vi "Rx Channel Config Page.vi"(8 "error in (no error)":errorcluster, 11 "Node Ptr":T1 format="%.0x") -> (0 "error out":errorcluster)   [LabVIEW 2016, in "UDP-Custom-Device System Explorer.lvlib"]
uses:
  UDP-Custom-Device System Explorer.lvlib
  <vilib>/NI Veristand/Custom Device API/Custom Device Item Ref.ctl
  <vilib>/NI VeriStand/Custom Device API/Custom Device API.lvlib
  Property Accessors/Shared Channel Accessors.lvlib
  <vilib>/NI VeriStand/Custom Device Tools/Custom Device Utility Library/Custom Device Utility Library.lvlib
panel:
  out "Imported Channel Configuration":i32[](listbox) caption="Channels"
  in  "Channel Configuration File":path
  in  "Description":string
  out "Name":string
  in  "SHDocVw.IWebBrowser":refnum<k7>(container)
  in  "General Header":cluster{"Section Name":string}={"Section Name"="Channel Configuration"}
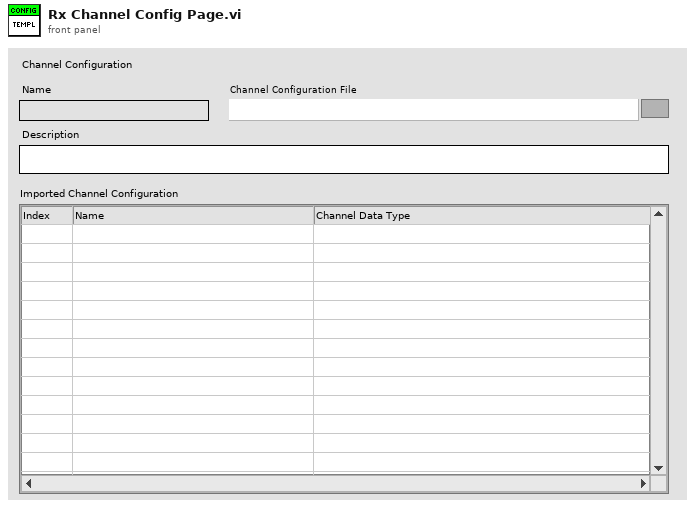
[diagram p1: front panel]
types:
  T1 = typedef "Custom Device API.lvlib/Custom Device Item Ref.ctl" = u64
  T2 = typedef "Custom Device API.lvlib/Custom Device Commands.ctl" = enum16{"Default", "Item renamed", "Shutdown", "Dynamic button pressed"}
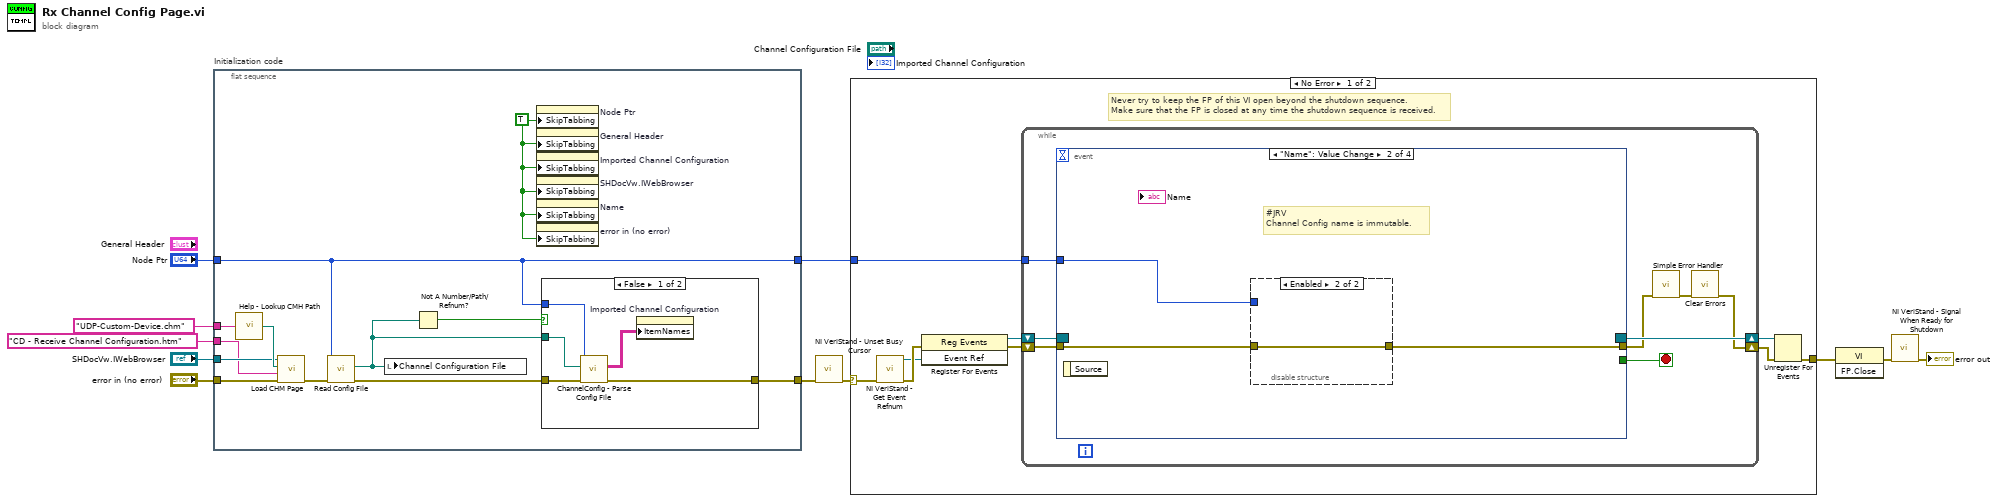
[diagram p0: block diagram]
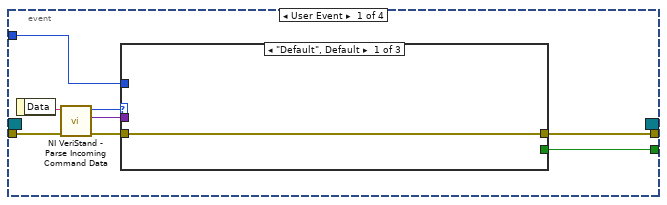
[diagram p3: hidden frame]
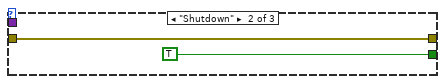
[diagram p4: hidden frame]
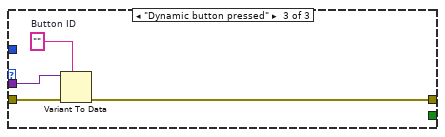
[diagram p5: hidden frame]
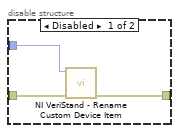
[diagram p6: hidden frame]
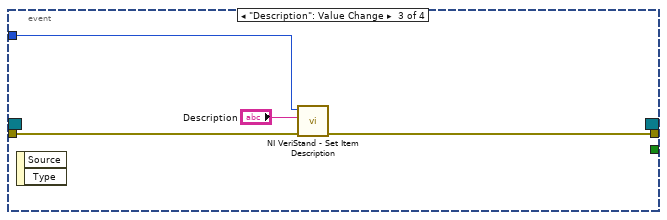
[diagram p7: hidden frame]
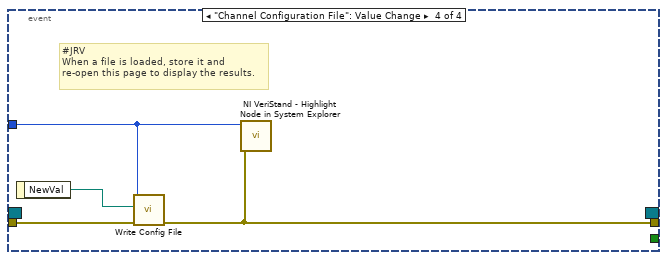
[diagram p8: hidden frame]
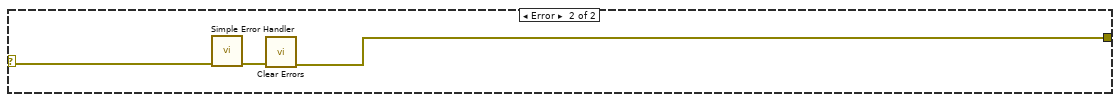
[diagram p9: hidden frame]
diagram:
  n1 = flat-sequence "Initialization code" {
    tunnel: "error in (no error)" -> [w22]
    tunnel: "Node Ptr" -> [w13]
    tunnel: [w17] -> w7
    tunnel: [w13] -> w4
    tunnel: "SHDocVw.IWebBrowser" -> [w21]
    tunnel: "CD - Receive Channel Configuration.htm" ("CD_CHM_Section") -> [w19]
    tunnel: "UDP-Custom-Device.chm" ("CD_CHM_FileName") -> [w20]
    frame #0 {
      w12 = TRUE ("Skip When Tabbing")
      n2 = call "Help - Lookup CMH Path.vi"("Main CMH File"=w20) -> ("Compiled CMH Path"=w23:path)
      n3 = call <vilib>:"Load CHM Page.vi"("error in (no error)"=w22, "HTML File"=w19, "Compiled CHM Path"=w23, "Web Browser Reference"=w21) -> ("error out"=w18:errorcluster)  [unwired: 7 in]
      n4 = call "Read Config File.vi"("error in (no error)"=w18, "Node Ptr"=w13) -> ("error out"=w16:errorcluster, "Config File"=w14:path)  [unwired: 7 in, 1 out]
      n5 = local write "Channel Configuration File"(w14) -> ()
      n6 = Not A Number/Path/Refnum?(number/path/refnum=w14) -> (NaN/Path/Refnum?=w15:bool)
      n7 = property on="Node Ptr" class="DigNum (strict)"("SkipTabbing"=w12) -> ()  [unwired: 2 in, 2 out]
      n8 = property on="General Header" class="Clust (strict)"("SkipTabbing"=w12) -> ()  [unwired: 2 in, 2 out]
      n9 = property on="Imported Channel Configuration" class="MCListbox (strict)"("SkipTabbing"=w12) -> ()  [unwired: 2 in, 2 out]
      n10 = property on="SHDocVw.IWebBrowser" class="AXCont"("SkipTabbing"=w12) -> ()  [unwired: 2 in, 2 out]
      n11 = property on="Name" class="Str"("SkipTabbing"=w12) -> ()  [unwired: 2 in, 2 out]
      n12 = property on="error in (no error)" class="Clust (strict)"("SkipTabbing"=w12) -> ()  [unwired: 2 in, 2 out]
      n13 = case shown="False" w15 {
        tunnel: [w25 w29] -> w17
        tunnel: w16 -> [w26 w29]
        tunnel: w14 -> [w28 _]
        tunnel: w13 -> [w27 _]
        frame False {
          n14 = call "ChannelConfig - Parse Config File.vi"("error in (no error)"=w26, "Config Path"=w28, "Node Ptr"=w27) -> ("error out"=w25:errorcluster, "Channel Configuration"=w24:string[][])  [unwired: 6 in, 1 out]
          n15 = property on="Imported Channel Configuration" class="MCListbox (strict)"("ItemNames"=w24) -> ()  [unwired: 2 in, 2 out]
        }
        frame True {
        }
      }
    }
  }
  n16 = call <vilib>:"NI VeriStand - Unset Busy Cursor.vi"("error in (no error)"=w7) -> ("error out"=w6:errorcluster)  [unwired: 10 out]
  n17 = case shown="No Error" w6 {
    selector: w6 -> [w30 w79]
    tunnel: [w35 w77] -> w11
    tunnel: w4 -> [w31 _]
    frame No Error {
      # "Never try to keep the FP of this VI open beyond the shutdown sequence.\nMake sure that the FP is closed at any time the shutdown sequence is received."
      n18 = call <vilib>:"NI VeriStand - Get Event Refnum.vi"("error in (no error)"=w30) -> ("error out"=w38:errorcluster, "Event Ref"=w34:refnum<user-event>)  [unwired: 9 out]
      n19 = register-events(error in=w38, w34) -> (reference out=w32:refnum<event-registration>, error out=w33:errorcluster)  [unwired: 1 in]
      n20 = while {
        tunnel: w31 -> [w42]
        shift-right: [w39] -> w36
        shift-left: w33 -> [w45]
        shift-right: [w46] -> w37
        shift-left: w32 -> [w44]
        stop <- w43 stop-if-true
        n21 = event shown="[1] \"Name\": Value Change" {
          selector: w44 -> [_ _ _ _]
          dyn-events: [_ _ _ _] -> w46
          timeout: _ -> [_ _ _ _]
          tunnel: w45 -> [w54 w64 w72 w74]
          tunnel: [w50 _ _ _] -> w43
          tunnel: [w49 w62 w69 w73] -> w41
          tunnel: w42 -> [w48 w63 w71 w76]
          event User Event {
            n22 = event-data() -> ("Data"=w53:string)  [unwired: 1 out]
            n23 = call <vilib>:"NI VeriStand - Parse Incoming Command Data.vi"("error in (no error)"=w54, "Incoming data"=w53) -> ("error out"=w52:errorcluster, "Outgoing data"=w47:variant, "Action"=w51:T2)  [unwired: 7 out]
            n24 = case shown="\"Default\", Default" w51 {
              tunnel: w52 -> [w55 w56 w61]
              tunnel: [_ TRUE _] -> w50
              tunnel: [w55 w56 w58] -> w49
              tunnel: w48 -> [_ _ _]
              tunnel: w47 -> [_ _ w60]
              frame "Default", Default {
              }
              frame "Shutdown" {
              }
              frame "Dynamic button pressed" {
                w59 = ""  # Button ID
                n25 = Variant To Data(error in=w61, type=w59, Variant=w60) -> (error out=w58:errorcluster)  [unwired: 1 out]
              }
            }
          }
          event "Name": Value Change {
            # "#JRV\nChannel Config name is immutable."
            n26 = event-data() -> ()  [unwired: 2 out]
            n27 = disable-structure shown="Enabled" {
              disable-tunnel: w64 -> [w67 w68]
              disable-tunnel: w63 -> [w66 _]
              disable-tunnel: [w65 w68] -> w62
              frame Disabled {
                n28 = call <vilib>:"NI VeriStand - Rename Custom Device Item.vi"("error in (no error)"=w67, "Item Ref in"=w66) -> ("error out"=w65:errorcluster)  [unwired: 7 in, 2 out]
              }
              frame Enabled {
              }
            }
          }
          event "Description": Value Change {
            n29 = event-data() -> ()  [unwired: 3 out]
            n30 = call <vilib>:"NI VeriStand - Set Item Description.vi"("error in (no error)"=w72, "Description"="Description", "Item Ref in"=w71) -> ("error out"=w69:errorcluster)  [unwired: 6 in, 2 out]
          }
          event "Channel Configuration File": Value Change {
            # "#JRV\nWhen a file is loaded, store it and\nre-open this page to display the results."
            n31 = event-data() -> ("NewVal"=w75:path)  [unwired: 1 out]
            n32 = call "Write Config File.vi"("error in (no error)"=w74, "Config File"=w75, "Node Ptr"=w76) -> ("error out"=w73:errorcluster)  [unwired: 7 in, 1 out]
            n33 = call <vilib>:"NI VeriStand - Highlight Node in System Explorer.vi"("error in (no error)"=w73, "Item Ref in"=w76) -> ()  [unwired: 8 in, 2 out]
          }
        }
        n34 = call <vilib>:"Simple Error Handler.vi"("error in (no error)"=w41) -> ("error out"=w40:errorcluster)  [unwired: 1 in, 7 out]
        n35 = call <vilib>:"Clear Errors.vi"("error in (no error)"=w40) -> ("error out"=w39:errorcluster)  [unwired: 1 in, 5 out]
      }
      n36 = Unregister For Events(event registration refnum=w37, error in=w36) -> (error out=w35:errorcluster)
    }
    frame Error {
      n37 = call <vilib>:"Simple Error Handler.vi"("error in (no error)"=w79) -> ("error out"=w78:errorcluster)  [unwired: 1 in, 7 out]
      n38 = call <vilib>:"Clear Errors.vi"("error in (no error)"=w78) -> ("error out"=w77:errorcluster)  [unwired: 1 in, 5 out]
    }
  }
  n39 = invoke class="VI" method="FP.Close"(error in=w11) -> (error out=w10:errorcluster)  [unwired: 2 in, 2 out]
  n40 = call <vilib>:"NI VeriStand - Signal When Ready for Shutdown.vi"("error in (no error)"=w10) -> ("error out"=→"error out":errorcluster)  [unwired: 10 out]
